vi "Write Pozycja.vi"(8 "error in (no error)":errorcluster, 10 "Position":T1, 11 "Boid in":refnum<class "Boid.lvclass">) -> (0 "error out":errorcluster, 3 "Boid out":refnum<class "Boid.lvclass">)   [LabVIEW 2014, in "Boid.lvclass"]
uses:
  Boid.lvclass
  Typedefs/Position.ctl
  Boid.lvclass/Boid.ctl
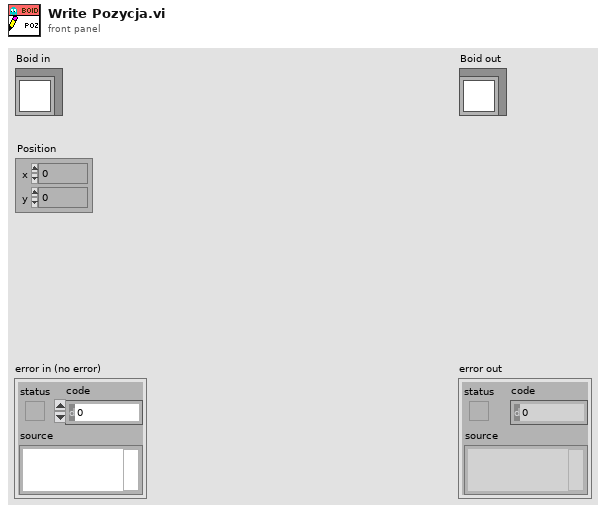
[diagram p1: front panel]
types:
  T1 = typedef "Position.ctl" = cluster{"x":i16, "y":i16}
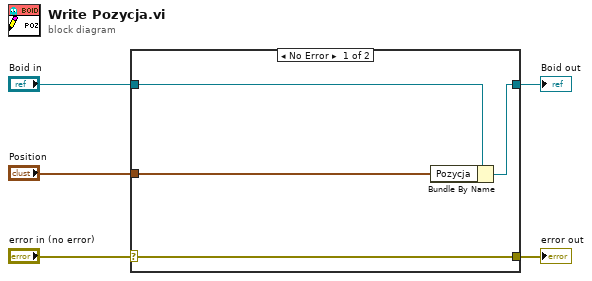
[diagram p0: block diagram]
diagram:
  n1 = case shown="No Error" "error in (no error)" {
    selector: "error in (no error)" -> [w9 w10]
    tunnel: [w9 w10] -> w4
    tunnel: [w7 w11] -> w2
    tunnel: "Boid in" -> [w8 w11]
    tunnel: "Position" -> [w6 _]
    frame No Error {
      n2 = Bundle By Name(cluster=w8, "Pozycja"=w6) -> (w7:refnum<class "Boid.lvclass">)
    }
    frame Error {
    }
  }
  "error out" <- w4
  "Boid out" <- w2
